vi "Get UDP Broadcast Reference.vi"(8 "error in (no error)":errorcluster, 9 "UDP Broadcast Link Timeout":i32=100) -> (0 "error out":errorcluster, 3 "Connection info out":T1)   [LabVIEW 2016, in "Assert API Components.lvlib" / "Log Assert Core.lvlib"]
doc: "Uses a single element queue to get and maintain a single instance UDP reference to broadcast the IP Address for all asserts on a single target. As long as the queue is in memory the reference should be valid. If the queue dies - the reference will be recreated."
uses:
  Log Assert Core.lvlib
  <vilib>/NI/STM/UDP/UDP Connection Info.ctl
  <vilib>/NI/STM/SubVIs/MetaDataElement.ctl
  <vilib>/NI/STM/UDP/UDP Read Options.ctl
  <vilib>/NI/STM/UDP/Read Meta Data (UDP Ref).vi
  <vilib>/NI/STM/UDP/Read Meta Data (UDP Clst).vi
  <vilib>/NI/STM/NI STM.lvlib
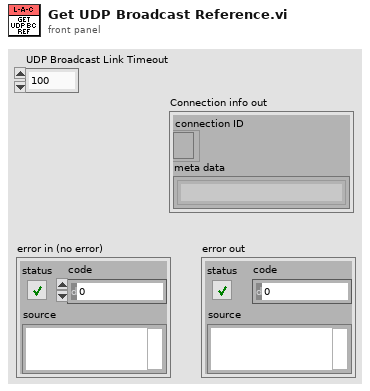
[diagram p1: front panel]
types:
  T1 = typedef "NI STM.lvlib/UDP Connection Info.ctl" = cluster{"connection ID":refnum<k16>, "meta data":T2[]}
  T2 = typedef "NI STM.lvlib/MetaDataElement.ctl" = string
  T3 = typedef "NI STM.lvlib/UDP Read Options.ctl" = cluster{"ignore timeout error":bool, "timeout ms (1000)":i32, "max size (548)":i32}
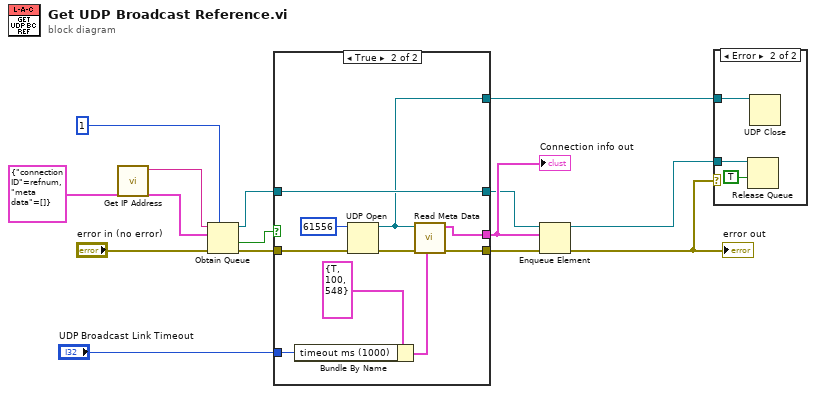
[diagram p0: block diagram]
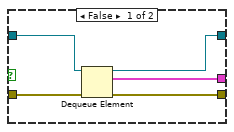
[diagram p3: hidden frame]
diagram:
  n1 = call "Get IP Address.vi"() -> ("IP Address"=w3:string)  [unwired: 11 in]
  n2 = Obtain Queue(max queue size (-1, unlimited)=1, name (unnamed)=w3, element data type=T1 {"connection ID"=refnum, "meta data"=[]} ("connection info out"), error in (no error)="error in (no error)") -> (queue out=w11:refnum<queue>, created new?=w10:bool, error out=w9:errorcluster)  [unwired: 1 in]
  n3 = case shown="True" w10 {
    tunnel: [w16 w24] -> w13
    tunnel: [w15 w25] -> w8
    tunnel: w9 -> [w19 w27]
    tunnel: w11 -> [w18 w26]
    tunnel: [w17 w26] -> w12
    tunnel: [_ w22] -> w2
    tunnel: "UDP Broadcast Link Timeout" -> [_ w20]
    frame False {
      n4 = Dequeue Element(queue=w18, error in (no error)=w19) -> (queue out=w17:refnum<queue>, element=w16:T1, error out=w15:errorcluster)  [unwired: 1 in, 1 out]
    }
    frame True {
      n5 = Bundle By Name(cluster=T3 {"ignore timeout error"=TRUE, "timeout ms (1000)"=100, "max size (548)"=548} ("options"), "timeout ms (1000)"=w20) -> (w21:T3)
      n6 = UDP Open(8:w27, 11:u16 61556 ("local port")) -> (port=w22:refnum<k16>, 0:w29:errorcluster)  [unwired: 3 in, 1 out]
      n7 = call-poly <vilib>:"Read Meta Data.vi"("options"=w21, "error in"=w29, "connection ID"=w22) -> ("error out"=w25:errorcluster, "connection info out"=w24:T1)  [unwired: 5 in, 2 out]
    }
  }
  "Connection info out" <- w13
  n8 = Enqueue Element(queue=w12, element=w13, error in (no error)=w8) -> (queue out=w4:refnum<queue>, error out=w5:errorcluster)  [unwired: 1 in, 1 out]
  "error out" <- w5
  n9 = case shown="Error" w5 {
    tunnel: w4 -> [_ w32]
    tunnel: w2 -> [_ w30]
    frame No Error {
    }
    frame Error {
      n10 = Release Queue(queue=w32, force destroy? (F)=TRUE) -> ()  [unwired: 1 in, 3 out]
      n11 = UDP Close(connection ID=w30) -> ()  [unwired: 1 in, 2 out]
    }
  }
